vi "Close Refs.vi"(8 "error in":errorcluster, 11 "PWM data(RT)":T1) -> (0 "error out":errorcluster)   [LabVIEW 2013, in "PWM Engine.lvlib"]
uses:
  PWM Engine.lvlib
  Shared/Types/PWM data(RT).ctl
  Shared/Types/PWM out info(RT).ctl
  Shared/Types/PWM in info(RT).ctl
  <vilib>/FPGAPlugInAG/Dynamic/niLvFpga_Close_Dynamic.vi
  <vilib>/rvi/interface/nirviCloseFPGA/nirviCloseFPGA.xnode
  Shared/PWM Shared.lvlib
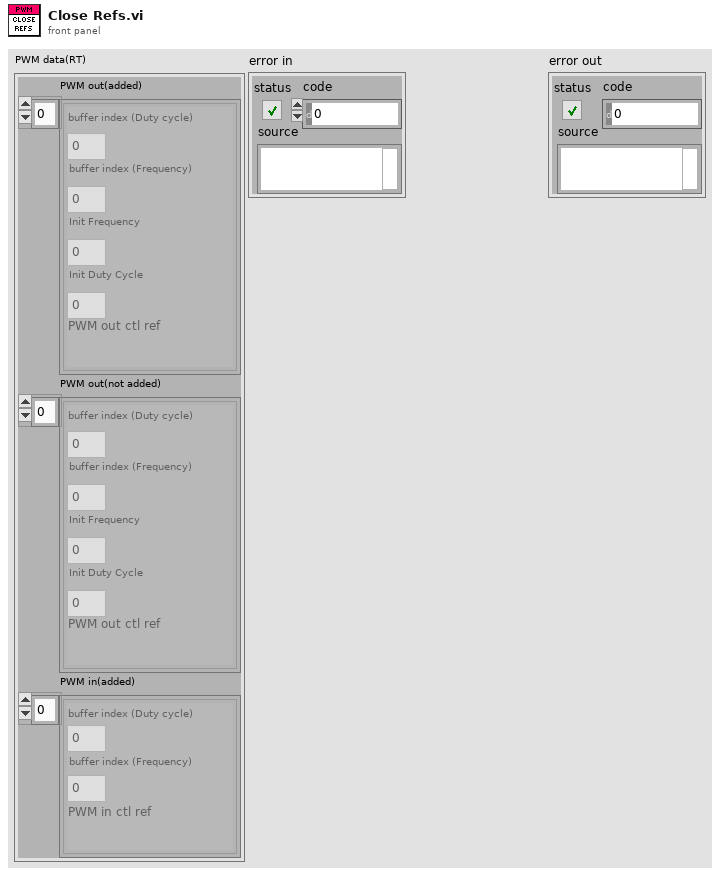
[diagram p1: front panel]
types:
  T1 = typedef "PWM Shared.lvlib/PWM data(RT).ctl" = cluster{"PWM out(added)":T2[], "PWM out(not added)":T2[], "PWM in(added)":T3[]}
  T2 = typedef "PWM Shared.lvlib/PWM out info(RT).ctl" = cluster{"buffer index (Duty cycle)":i32, "buffer index (Frequency)":i32, "Init Frequency":dbl, "Init Duty Cycle":dbl, "PWM out ctl ref":refnum<k20>}
  T3 = typedef "PWM Shared.lvlib/PWM in info(RT).ctl" = cluster{"buffer index (Duty cycle)":i32, "buffer index (Frequency)":i32, "PWM in ctl ref":refnum<k20>}
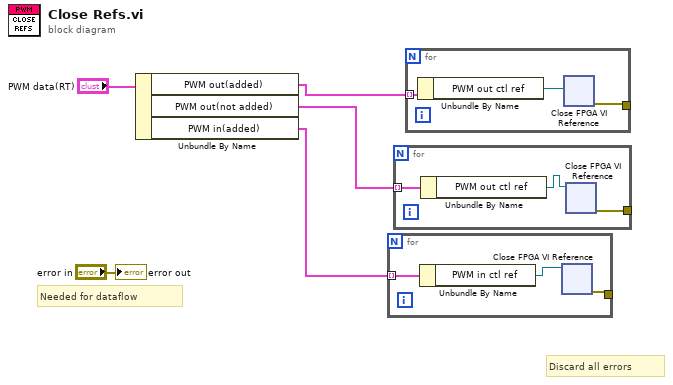
[diagram p0: block diagram]
diagram:
  # "Needed for dataflow"
  # "Discard all errors"
  n1 = Unbundle By Name("PWM data(RT)") -> ("PWM out(added)"=w2:T2[], "PWM out(not added)"=w4:T2[], "PWM in(added)"=w3:T3[])
  n2 = for {
    tunnel: w3 -> [w8] mode=indexing
    tunnel: [w6] -> _
    n3 = Unbundle By Name(w8) -> ("PWM in ctl ref"=w7:refnum<k20>)
    n4 = xnode "Close FPGA VI Reference"("FPGA VI Reference In"=w7) -> ("error out"=w6:errorcluster)  [unwired: 1 in]
  }
  n5 = for {
    tunnel: w4 -> [w11] mode=indexing
    tunnel: [w9] -> _
    n6 = Unbundle By Name(w11) -> ("PWM out ctl ref"=w10:refnum<k20>)
    n7 = xnode "Close FPGA VI Reference"("FPGA VI Reference In"=w10) -> ("error out"=w9:errorcluster)  [unwired: 1 in]
  }
  n8 = for {
    tunnel: w2 -> [w14] mode=indexing
    tunnel: [w12] -> _
    n9 = Unbundle By Name(w14) -> ("PWM out ctl ref"=w13:refnum<k20>)
    n10 = xnode "Close FPGA VI Reference"("FPGA VI Reference In"=w13) -> ("error out"=w12:errorcluster)  [unwired: 1 in]
  }
  "error out" <- "error in"
